vi "List Policy Principals.vi"(8 "error in (no error)":errorcluster, 10 "Policy":string, 11 "IoT Session in":refnum<class "IoT Session.lvclass">) -> (0 "error out":errorcluster, 2 "Policy Principals":string[](array[string]), 3 "IoT Session out":refnum<class "IoT Session.lvclass">)   [LabVIEW 2015, in "NI_AWS_IoT.lvlib" / "IoT Session.lvclass"]
uses:
  IoT Session.lvclass
  Core/HTTP Request/Request Options.ctl
  Core/HTTP Request/Name Value Pair.ctl
  Core/HTTP Request/Region handling.ctl
  Core/HTTP Request/URL formatting.ctl
  Core/HTTP Request/HTTP Request.lvclass
  JSON Parsing/NI_JSON Parsing.lvlib
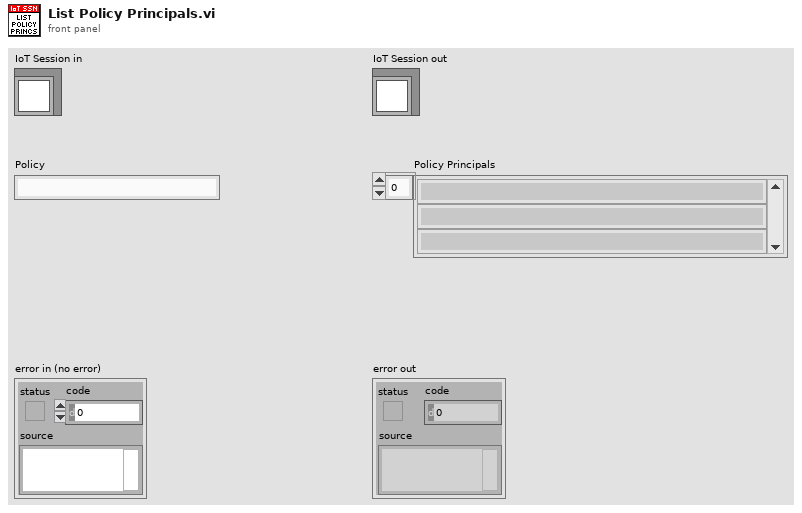
[diagram p1: front panel]
types:
  T1 = typedef "NI_AWS_Core.lvlib/HTTP Request.lvclass/Name Value Pair.ctl" = cluster{"name":string, "value":string}
  T2 = typedef "NI_AWS_Core.lvlib/HTTP Request.lvclass/Request Options.ctl" = cluster{"request headers":T1[], "request parameters":T1[], "request body":string, "region handling":T3, "URL formatting":T4}
  T3 = typedef "NI_AWS_Core.lvlib/HTTP Request.lvclass/Region handling.ctl" = enum16{"use region everywhere", "use region (authentication only)", "use region (URL only)", "ignore region everwhere"}
  T4 = typedef "NI_AWS_Core.lvlib/HTTP Request.lvclass/URL formatting.ctl" = enum16{"region-", "region."}
  T5 = typedef "NI_AWS_Core.lvlib/HTTP Request.lvclass/Response.ctl" = cluster{"Headers":string, "Body":string}
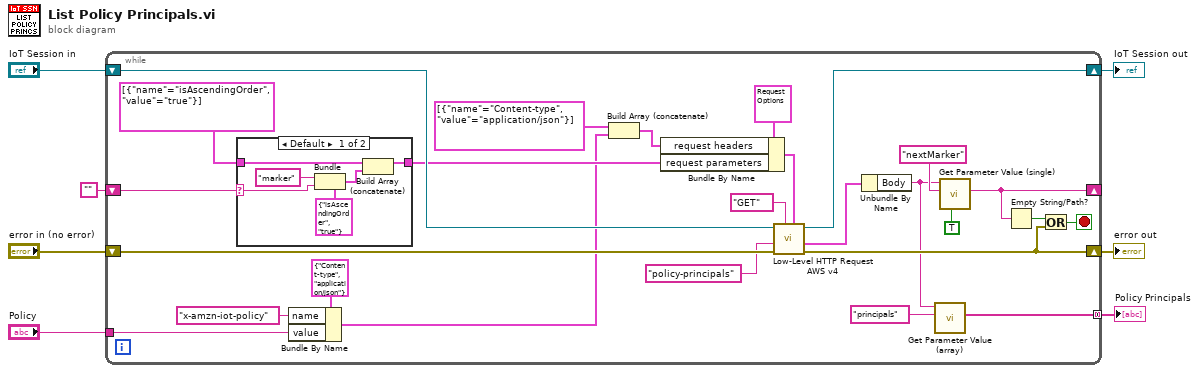
[diagram p0: block diagram]
diagram:
  n1 = while {
    shift-right: [w21] -> w6
    shift-left: "error in (no error)" -> [w30]
    shift-right: [w29] -> w5
    shift-left: "IoT Session in" -> [w28]
    shift-right: [w23] -> _
    shift-left: "" -> [w25]
    tunnel: [w9] -> w2 mode=concatenating
    tunnel: "Policy" -> [w11]
    stop <- w20 stop-if-true
    n2 = case shown="Default" w25 {
      selector: w25 -> [w35 _]
      tunnel: T1[] [{"name"="isAscendingOrder", "value"="true"}] ("request parameters") -> [w39 w40]
      tunnel: [w38 w40] -> w15
      frame Default {
        n3 = Bundle(cluster=T1 {"name"="isAscendingOrder", "value"="true"} ("Name Value Pair"), "name"="marker", "value"=w35) -> (w36:T1)
        n4 = Build Array (concatenate)(w39, w36) -> (w38:T1[])
      }
      frame "" {
      }
    }
    n5 = Bundle By Name(cluster=T1 {"name"="Content-type", "value"="application/json"} ("Cluster"), "name"="x-amzn-iot-policy", "value"=w11) -> (w10:T1)
    n6 = Build Array (concatenate)(T1[] [{"name"="Content-type", "value"="application/json"}] ("request headers"), w10) -> (w14:T1[])
    n7 = Bundle By Name(cluster=T2 {"request headers"=[], "request parameters"=[], "request body"="", "region handling"=enum."use region everywhere", "URL formatting"=enum."region."} ("Request Options"), "request headers"=w14, "request parameters"=w15) -> (w31:T2)
    n8 = call "Low-Level HTTP Request AWS v4.vi"("Request Options"=w31, "HTTP-Verb"="GET", "error in (no error)"=w30, "URL Suffix"="policy-principals" ("string"), "AWS Core in"=w28) -> ("error out"=w21:errorcluster, "Response"=w26:T5, "AWS Core out"=w29:refnum<class "IoT Session.lvclass">)  [unwired: 3 in, 1 out]
    n9 = Unbundle By Name(w26) -> ("Body"=w8:string)
    n10 = call "Get Parameter Value (array).vi"("Parameter Name"="principals", "JSON"=w8) -> ("Parameter Values"=w9:string[])  [unwired: 7 in, 2 out]
    n11 = call "Get Parameter Value (single).vi"("Clear Null"=TRUE, "Parameter Name"="nextMarker", "JSON"=w8) -> ("Parameter Value"=w23:string)  [unwired: 5 in, 3 out]
    n12 = Empty String/Path?(string/path=w23) -> (empty?=w22:bool)
    n13 = Or(x=w22, y=w21) -> (x .or. y?=w20:bool)
  }
  "error out" <- w6
  "IoT Session out" <- w5
  "Policy Principals" <- w2
